vi "NI-XNET Monitor Get Comm State.vi"(8 "Error In":errorcluster, 11 "Process  Data In":T1) -> (0 "Error Out":errorcluster, 3 "Process  Data Out":T1)   [LabVIEW 2018, in "NI-XNET Monitor Engine.lvlib"]
uses:
  NI-XNET Monitor Engine.lvlib
  RTMonitorRefnums.ctl
  <vilib>/NI/NIVS Inline Async API/_Data Access Engine/Data Access Engine/Types/Write.DVR.ctl
  <vilib>/NI/NIVS Inline Async API/_Data Access Engine/Access Type Classes/Write/Write.lvclass
  <vilib>/NI/NIVS Inline Async API/_Data Access Engine/Access Type Classes/Write/Write.lvclass/Write.ctl
  <vilib>/NI/NIVS Inline Async API/_Data Access Engine/Data Access Engine/Methods/Write.Data.vi
  <vilib>/NI/NIVS Inline Async API/_Data Access Engine/Access Type Classes/Write/Write.ProcessData.vi
  <vilib>/xnet/xnet.llb/XNET Read (Frame LIN).vi
  <vilib>/xnet/xnet.llb/XNET Read (State LIN Comm).vi
  <vilib>/xnet/xnet.llb/XNET Read (Frame FlexRay).vi
  <vilib>/xnet/xnet.llb/XNET Read (State FlexRay Comm).vi
  <vilib>/xnet/xnet.llb/XNET Read (Frame CAN).vi
  <vilib>/xnet/xnet.llb/XNET Read (State CAN Comm).vi
  <vilib>/NI/NIVS Inline Async API/_Data Access Engine/Data Access Engine/Data Access Engine.lvclass
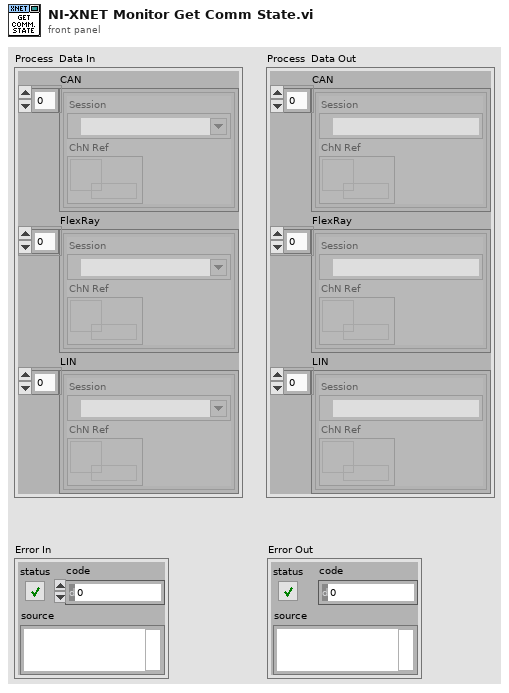
[diagram p1: front panel]
types:
  T1 = typedef "NI-XNET Monitor Engine.lvlib/RTMonitorRefnums.ctl" = cluster{"CAN":cluster{"Session":refnum<k21>, "ChN Ref":T2}[], "FlexRay":cluster{"Session":refnum<k21>, "ChN Ref":T2}[], "LIN":cluster{"Session":refnum<k21>, "ChN Ref":T2}[]}
  T2 = typedef "Data Access Engine.lvlib/Data Access Engine.lvclass/Write.DVR.ctl" = refnum<data-value>
  T3 = typedef "XNET Frame FlexRay.ctl" = cluster{"timestamp":timestamp, "payload":u8[], "slot":u16, "type":T4, "cycle count":u8, "startup?":bool, "sync?":bool, "preamble?":bool, "ch A":bool, "ch B":bool, "echo?":bool}
  T4 = typedef "XNET Frame Type FlexRay.ctl" = u8
  T5 = typedef "XNET FlexRay Comm.ctl" = cluster{"fault code":i32, "fault?":bool, "FlexRay POC state":T6, "clock correction failed":u8, "passive to active count":u8, "channel A sleep?":bool, "channel B sleep?":bool}
  T6 = typedef "XNET FlexRay POC State.ctl" = u8
  T7 = typedef "XNET Frame CAN.ctl" = cluster{"timestamp":timestamp, "payload":u8[], "identifier":u32, "type":T8, "extended?":bool, "echo?":bool}
  T8 = typedef "XNET Frame Type CAN.ctl" = u8
  T9 = typedef "XNET CAN Comm.ctl" = cluster{"fault code":i32, "fault?":bool, "communication state":T10, "last error":T11, "receive error counter":u8, "transmit error counter":u8, "transceiver error?":bool, "sleep?":bool}
  T10 = typedef "XNET CAN Comm State.ctl" = u8
  T11 = typedef "XNET CAN Last Err.ctl" = u8
  T12 = typedef "XNET Frame LIN.ctl" = cluster{"timestamp":timestamp, "payload":u8[], "identifier":u32, "type":T13, "event ID":u8, "event slot?":bool, "echo?":bool}
  T13 = typedef "XNET Frame Type LIN.ctl" = u8
  T14 = typedef "XNET LIN Comm.ctl" = cluster{"fault code":i32, "fault?":bool, "communication state":T15, "last error":T16, "last error received":u8, "last error expected":u8, "last error identifier":u8, "sleep?":bool, "transceiver ready?":bool, "schedule index":u8}
  T15 = typedef "XNET LIN Comm State.ctl" = u8
  T16 = typedef "XNET LIN Last Err.ctl" = u8
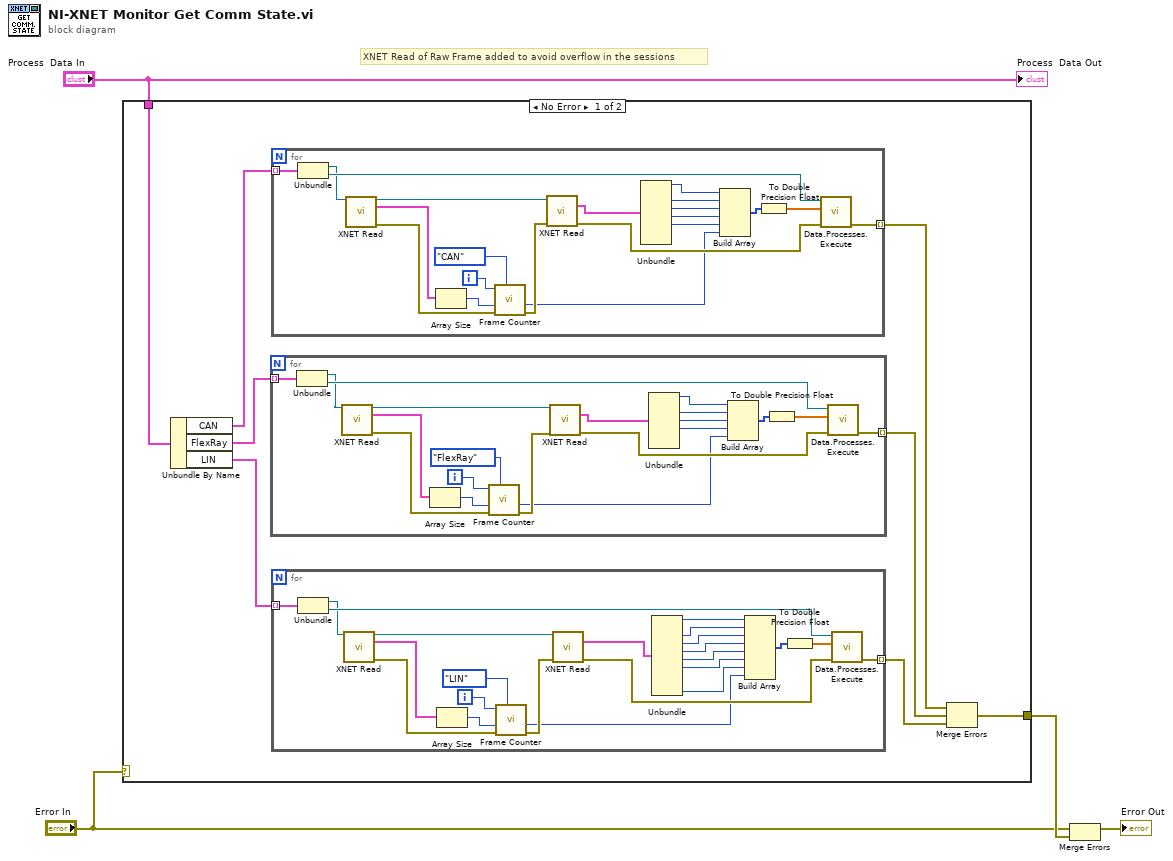
[diagram p0: block diagram]
diagram:
  # "XNET Read of Raw Frame added to avoid overflow in the sessions"
  n1 = case shown="No Error" "Error In" {
    tunnel: "Process  Data In" -> [w12 _]
    tunnel: [w5 _] -> w2
    frame No Error {
      n2 = Unbundle By Name(w12) -> ("CAN"=w11:cluster{"Session":refnum<k21>, "ChN Ref":T2}[], "FlexRay"=w10:cluster{"Session":refnum<k21>, "ChN Ref":T2}[], "LIN"=w6:cluster{"Session":refnum<k21>, "ChN Ref":T2}[])
      n3 = for {
        tunnel: w10 -> [w55] mode=indexing
        tunnel: [w51] -> w8 mode=indexing
        i -> [w38]
        n4 = Unbundle(w55) -> ("Session"=w44:refnum<k21>, "ChN Ref"=w50:T2)
        n5 = call-poly <vilib>:"XNET Read.vi"("session in"=w44) -> ("session out"=w43:refnum<k21>, "data"=w39:T3[], "error out"=w40:errorcluster)  [unwired: 11 in, 1 out]
        n6 = Array Size(array=w39) -> (size(s)=w42:i32)
        n7 = call "Frame Counter.vi"("bus type"=enum16{"CAN", "FlexRay", "LIN"}."FlexRay", "error in (no error)"=w40, "new frames"=w42, "bus index (bus count for init)"=w38) -> ("error out"=w41:errorcluster, "total frames"=w37:u32)  [unwired: 6 in]
        n8 = call-poly <vilib>:"XNET Read.vi"("session in"=w43, "error in (no error)"=w41) -> ("FlexRay comm"=w54:T5, "error out"=w46:errorcluster)  [unwired: 11 in, 1 out]
        n9 = Unbundle(w54) -> ("fault code"=w53:i32, "FlexRay POC state"=w49:T6, "clock correction failed"=w48:u8, "passive to active count"=w47:u8)  [unwired: 3 out]
        n10 = Build Array(w53, w49, w48, w47, w37) -> (w52:u32[])
        n11 = To Double Precision Float(number=w52) -> (double precision float=w45:dbl[])
        n12 = call-poly <vilib>:"Data.Processes.Execute.vi"("error in (no error)"=w46, "Values"=w45, "Ref"=w50) -> ("error out"=w51:errorcluster)  [unwired: 8 in]
      }
      n13 = for {
        tunnel: w11 -> [w76] mode=indexing
        tunnel: [w74] -> w7 mode=indexing
        i -> [w58]
        n14 = Unbundle(w76) -> ("Session"=w72:refnum<k21>, "ChN Ref"=w73:T2)
        n15 = call-poly <vilib>:"XNET Read.vi"("session in"=w72) -> ("session out"=w65:refnum<k21>, "data"=w60:T7[], "error out"=w62:errorcluster)  [unwired: 11 in, 1 out]
        n16 = Array Size(array=w60) -> (size(s)=w59:i32)
        n17 = call "Frame Counter.vi"("bus type"=enum16{"CAN", "FlexRay", "LIN"}."CAN", "error in (no error)"=w62, "new frames"=w59, "bus index (bus count for init)"=w58) -> ("error out"=w61:errorcluster, "total frames"=w57:u32)  [unwired: 6 in]
        n18 = call-poly <vilib>:"XNET Read.vi"("session in"=w65, "error in (no error)"=w61) -> ("CAN comm"=w64:T9, "error out"=w63:errorcluster)  [unwired: 11 in, 1 out]
        n19 = Unbundle(w64) -> ("fault code"=w67:i32, "communication state"=w71:T10, "last error"=w70:T11, "receive error counter"=w69:u8, "transmit error counter"=w68:u8)  [unwired: 3 out]
        n20 = Build Array(w67, w71, w70, w69, w68, w57) -> (w75:u32[])
        n21 = To Double Precision Float(number=w75) -> (double precision float=w66:dbl[])
        n22 = call-poly <vilib>:"Data.Processes.Execute.vi"("error in (no error)"=w63, "Values"=w66, "Ref"=w73) -> ("error out"=w74:errorcluster)  [unwired: 8 in]
      }
      n23 = for {
        tunnel: w6 -> [w35] mode=indexing
        tunnel: [w31] -> w9 mode=indexing
        i -> [w13]
        n24 = Unbundle(w35) -> ("Session"=w20:refnum<k21>, "ChN Ref"=w29:T2)
        n25 = call-poly <vilib>:"XNET Read.vi"("session in"=w20) -> ("session out"=w21:refnum<k21>, "data"=w15:T12[], "error out"=w16:errorcluster)  [unwired: 11 in, 1 out]
        n26 = Array Size(array=w15) -> (size(s)=w19:i32)
        n27 = call "Frame Counter.vi"("bus type"=enum16{"CAN", "FlexRay", "LIN"}."LIN", "error in (no error)"=w16, "new frames"=w19, "bus index (bus count for init)"=w13) -> ("error out"=w17:errorcluster, "total frames"=w14:u32)  [unwired: 6 in]
        n28 = call-poly <vilib>:"XNET Read.vi"("session in"=w21, "error in (no error)"=w17) -> ("LIN comm"=w34:T14, "error out"=w30:errorcluster)  [unwired: 11 in, 1 out]
        n29 = Unbundle(w34) -> ("fault code"=w33:i32, "communication state"=w28:T15, "last error"=w27:T16, "last error received"=w26:u8, "last error expected"=w25:u8, "last error identifier"=w24:u8, "schedule index"=w23:u8)  [unwired: 3 out]
        n30 = Build Array(w33, w28, w27, w26, w25, w24, w23, w14) -> (w32:u32[])
        n31 = To Double Precision Float(number=w32) -> (double precision float=w22:dbl[])
        n32 = call-poly <vilib>:"Data.Processes.Execute.vi"("error in (no error)"=w30, "Values"=w22, "Ref"=w29) -> ("error out"=w31:errorcluster)  [unwired: 8 in]
      }
      n33 = Merge Errors(w7, w8, w9) -> (w5:errorcluster)
    }
    frame Error {
    }
  }
  n34 = Merge Errors("Error In", w2) -> (→"Error Out":errorcluster)
  "Process  Data Out" <- "Process  Data In"
